vi "Util_Convert U32 to HexString.vi"(7 "Number":u32, 13 "Min Width":i16) -> (8 "HexString":string)   [LabVIEW 2023]
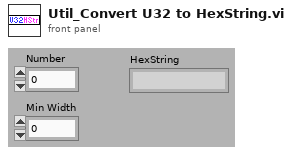
[diagram p1: front panel]
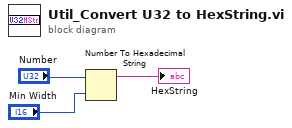
[diagram p0: block diagram]
diagram:
  n1 = Number To Hexadecimal String(1:"Min Width", 2:"Number") -> (0:→"HexString":string)
